vi "Calcu_Comp_Tens.vi"(8 "error in":errorcluster caption="에러 입력(에러 없음)", 9 "클러스터":T1, 10 "Condition set":string[][][](array[string]), 11 "Func_ext":string) -> (0 "error out":errorcluster caption="에러 출력", 1 "단 번호":i32, 2 "Resolution":string[][][](array[string]), 3 "Spec Out":string[][][](array[string]), 4 "ItemNames 출력":string[][](array[string]), 5 "condition out":string[][][](array[string]), 6 "cmc out":string[][][](array[string]), 7 "Spec Default":string[][][](array[string]))   [LabVIEW 2020]
uses:
  Controls/Cmd_Var Data IO.ctl
  Public/Polymorph/Data Class_2D Str.vi
  Public/Polymorph/Rmv Empt Arr_2D Str.vi
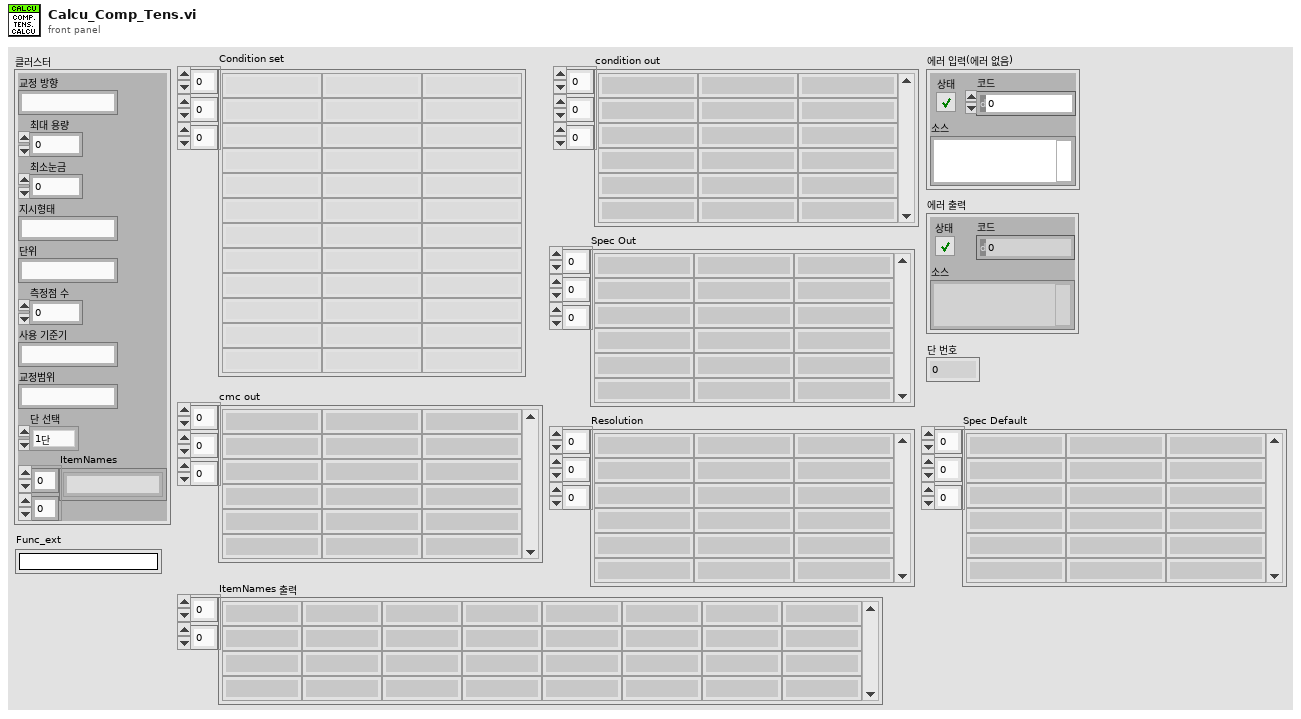
[diagram p1: front panel]
types:
  T1 = cluster{"교정 방향":string, "최대 용량":dbl, "최소눈금":dbl, "지시형태":string, "단위":string, "측정점 수":u8, "사용 기준기":string, "교정범위":string, "단 선택":enum8{"1단", "2단", "3단", "4단", "5단", "6단", "7단", "8단", "9단", "10단"}, "ItemNames":string[][]}
  T2 = typedef "Cmd_Var Data IO.ctl" = enum16{"Condition", "Condition Default", "Condition_Temp", "Resolution", "Resolution Default", "Resolution Old", "Spec", "Spec Default", "Spec Old", "Spec Temp", "Result", "Result2", "Result3", "Result_Temp", "Result_ADJ", "Result_ADJ2", "STD1", "STD2", "STD3", "STD4", "STD5", "STD Temp", "CMC", "CMC Default"}
  T3 = enum8{"1단", "2단", "3단", "4단", "5단", "6단", "7단", "8단", "9단", "10단"}
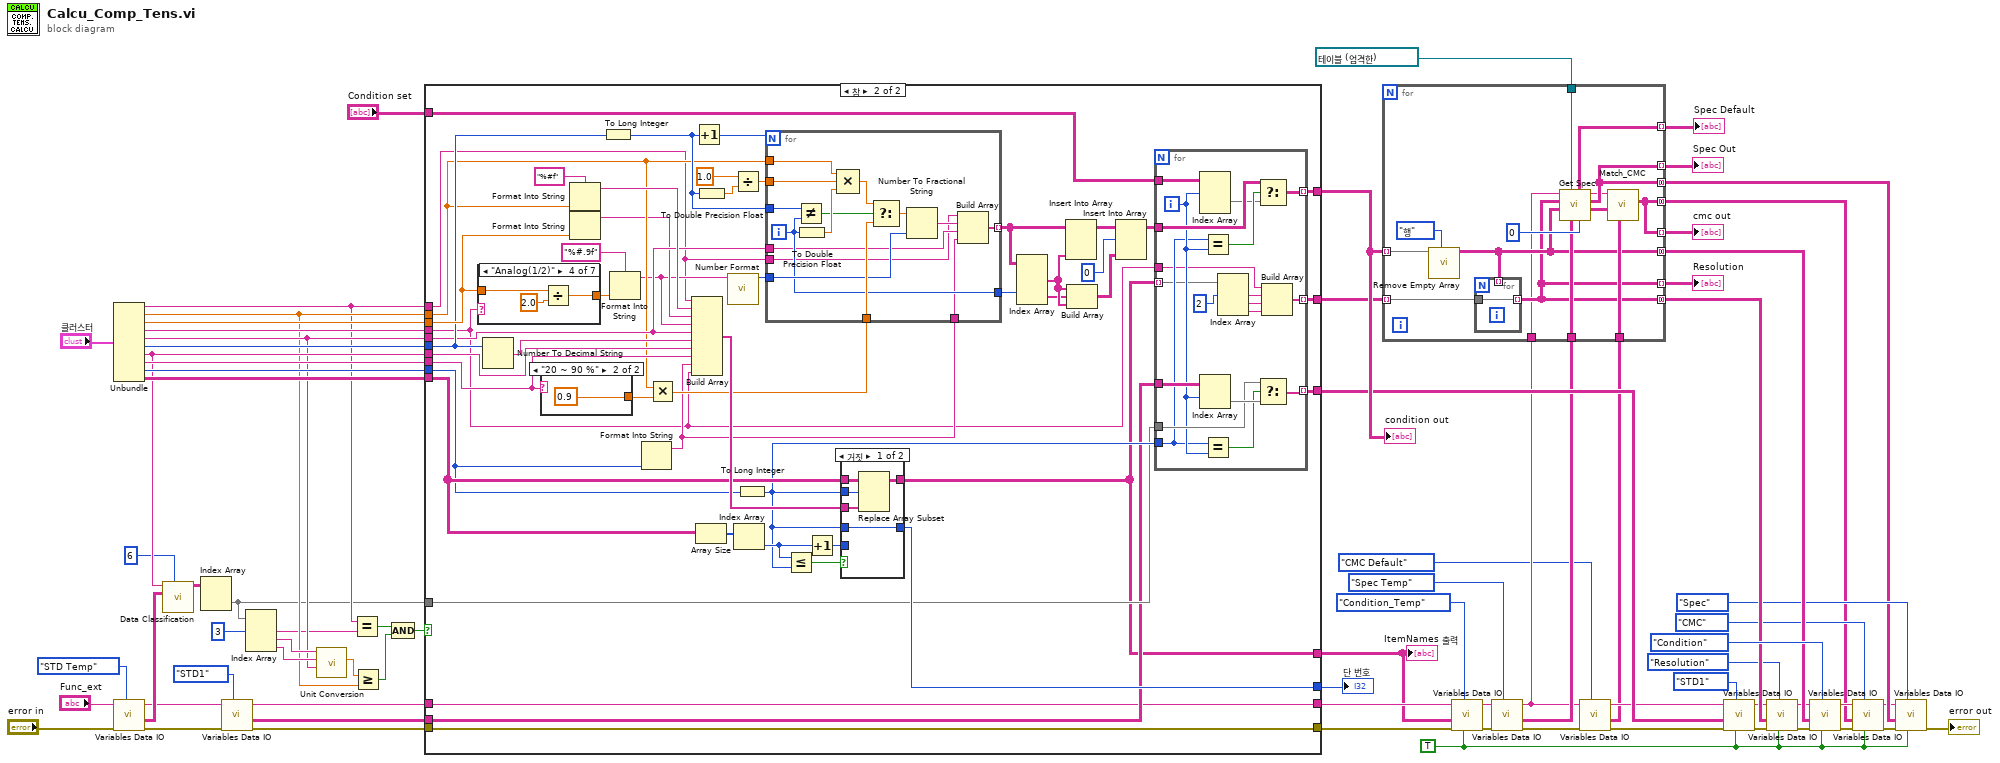
[diagram p0: block diagram]
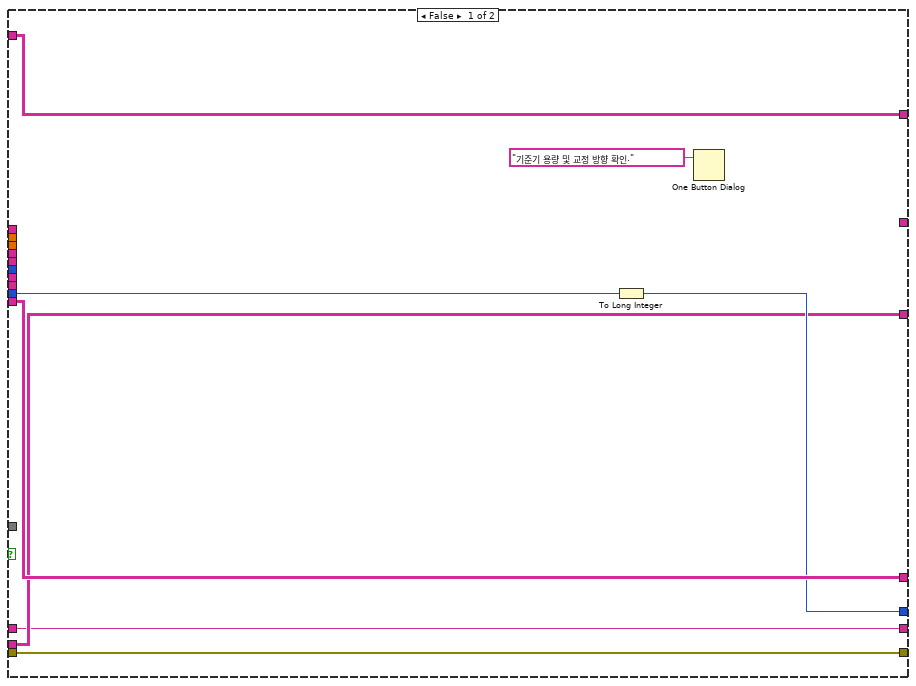
[diagram p2: hidden frame]
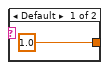
[diagram p3: hidden frame]
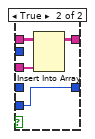
[diagram p4: hidden frame]
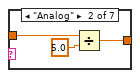
[diagram p6: hidden frame]
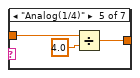
[diagram p8: hidden frame]
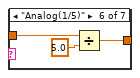
[diagram p9: hidden frame]
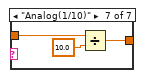
[diagram p10: hidden frame]
diagram:
  w2 = TRUE ("Write blank data ?(T)")
  n1 = Unbundle("클러스터") -> ("교정 방향"=w58:string, "최대 용량"=w60:dbl, "최소눈금"=w74:dbl, "지시형태"=w73:string, "단위"=w62:string, "측정점 수"=w70:u8, "사용 기준기"=w67:string, "교정범위"=w69:string, "단 선택"=w71:T3, "ItemNames"=w72:string[][])
  n2 = call "Variables Data IO.vi"("Select"=Cmd_Var_Data_IO."STD Temp", "error in"="error in", "Func_ext"="Func_ext") -> ("error out"=w44:errorcluster, "Data Out"=w46:string[][], "Func_ext Out"=w43:string)  [unwired: 6 in]
  n3 = call-poly "Data Classification.vi"("인덱스"=6, "DATA 입력"=w46, "검색 문자열"=w67) -> ("DATA 출력"=w66:string[][])  [unwired: 4 in, 4 out]
  n4 = Index Array(array=w66) -> (element=w53:string[])  [unwired: 2 in]
  n5 = call "Variables Data IO.vi"("Select"=Cmd_Var_Data_IO."STD1", "error in"=w44, "Func_ext"=w43) -> ("error out"=w38:errorcluster, "Data Out"=w41:string[][], "Func_ext Out"=w35:string)  [unwired: 6 in]
  n6 = Index Array(array=w53, index #1=3 ("인덱스")) -> (element #1=w59:string, element #2=w64:string, element #3=w63:string)  [unwired: 2 in]
  n7 = call "Unit Conversion.vi"("환산단위"=w62, "입력단위"=w63, "입력값"=w64) -> ("환산값 (DBL)"=w61:dbl)  [unwired: 3 in, 5 out]
  n8 = Equal?(x=w58, y=w59) -> (x = y?=w57:bool)
  n9 = Greater Or Equal?(x=w61, y=w60) -> (x >= y?=w56:bool)
  n10 = Compound Arithmetic op=AND(w57, w56) -> (w54:bool)
  n11 = case shown="참" w54 {
    tunnel: w74 -> [_ w126]
    tunnel: w73 -> [_ w84]
    tunnel: w72 -> [w82 w124]
    tunnel: w71 -> [w81 w86]
    tunnel: w70 -> [_ w123]
    tunnel: w69 -> [_ w122]
    tunnel: [w80 w106] -> w68
    tunnel: [w83 w104] -> w51
    tunnel: [w82 w89] -> w3
    tunnel: w67 -> [_ w101]
    tunnel: w62 -> [_ w100]
    tunnel: w60 -> [_ w99]
    tunnel: w58 -> [_ w87]
    tunnel: w53 -> [_ w97]
    tunnel: "Condition set" -> [w83 w98]
    tunnel: w41 -> [w79 w96]
    tunnel: [w79 w95] -> w39
    tunnel: [w77 w92] -> w8
    tunnel: w35 -> [w77 w92]
    tunnel: [w76 w93] -> w7
    tunnel: w38 -> [w76 w93]
    tunnel: [_ w88] -> w34
    frame False {
      n12 = To Long Integer(number=w81) -> (32bit integer=w80:i32)
      n13 = One Button Dialog(message="기준기 용량 및 교정 방향 확인." ("메시지")) -> ()  [unwired: 1 in, 1 out]
    }
    frame True {
      w133 = "%#f" ("포맷 문자열")
      n14 = case shown="\"Analog(1/2)\"" w84 {
        tunnel: w126 -> [w179 w182 w183 w186 w189 w192 w195]
        tunnel: [w179 w180 w183 w184 w187 w190 w193] -> w129
        frame Default {
        }
        frame "Analog" {
          n15 = Divide(x=w182, y=5.0) -> (x/y=w180:dbl)
        }
        frame "Analog(1/1)" {
        }
        frame "Analog(1/2)" {
          n16 = Divide(x=w186, y=2.0) -> (x/y=w184:dbl)
        }
        frame "Analog(1/4)" {
          n17 = Divide(x=w189, y=4.0) -> (x/y=w187:dbl)
        }
        frame "Analog(1/5)" {
          n18 = Divide(x=w192, y=5.0) -> (x/y=w190:dbl)
        }
        frame "Analog(1/10)" {
          n19 = Divide(x=w195, y=10.0) -> (x/y=w193:dbl)
        }
      }
      n20 = Number To Decimal String(number=w123) -> (decimal integer string=w130:string)  [unwired: 1 in]
      n21 = case shown="\"20 ~ 90 %\"" w122 {
        tunnel: [1.0 0.9] -> w120
        frame Default {
        }
        frame "20 ~ 90 %" {
        }
      }
      n22 = Format Into String(format string=w133, w99) -> (resulting string=w127:string)  [unwired: 2 in, 1 out]
      n23 = Format Into String(format string=w133, w126) -> (resulting string=w91:string)  [unwired: 2 in, 1 out]
      n24 = To Long Integer(number=w123) -> (32bit integer=w115:i32)
      n25 = Format Into String(format string="%#.9f" ("포맷 문자열"), w129) -> (resulting string=w90:string)  [unwired: 2 in, 1 out]
      n26 = Format Into String(w86) -> (resulting string=w85:string)  [unwired: 3 in, 1 out]
      n27 = Multiply(x=w99, y=w120) -> (x*y=w119:dbl)
      n28 = Build Array(w87, w127, w91, w90, w100, w130, w101, w122, w85, w84) -> (w131:string[])
      n29 = Increment(x=w115) -> (x+1=w121:i32)
      n30 = Array Size(array=w124) -> (size(s)=w132:i32[])
      n31 = To Double Precision Float(number=w115) -> (double precision float=w116:dbl)
      n32 = call "Number Format.vi"("입력값"=w90) -> ("정밀도(단위적용)"=w118:i32)  [unwired: 10 in]
      n33 = Divide(x=1.0, y=w116) -> (x/y=w114:dbl)
      n34 = Index Array(array=w132) -> (element=w125:i32)  [unwired: 1 in]
      n35 = To Long Integer(number=w86) -> (32bit integer=w103:i32)
      n36 = for {
        N: w121 -> [_]
        tunnel: [w160] -> w113 mode=indexing
        tunnel: w99 -> [w168]
        tunnel: w115 -> [w167]
        tunnel: w119 -> [w166]
        tunnel: w118 -> [w161]
        tunnel: w114 -> [w162]
        tunnel: w100 -> [w157]
        tunnel: [w158] -> w94
        tunnel: w87 -> [w156]
        tunnel: w85 -> [w155]
        i -> [w158]
        n37 = Not Equal?(x=w167, y=w158) -> (x != y?=w165:bool)
        n38 = To Double Precision Float(number=w158) -> (double precision float=w169:dbl)
        n39 = Compound Arithmetic op=MULTIPLY(w168, w162, w169) -> (w164:dbl)
        n40 = Select(t=w164, s=w165, f=w166) -> (s? t:f=w159:dbl)
        n41 = Number To Fractional String(number=w159, precision (6)=w161) -> (F-format string=w163:string)  [unwired: 2 in]
        n42 = Build Array(w156, w163, w157, w155) -> (w160:string[])
      }
      n43 = Less Or Equal?(x=w125, y=w103) -> (x <= y?=w107:bool)
      n44 = Increment(x=w125) -> (x+1=w105:i32)
      n45 = case shown="거짓" w107 {
        tunnel: [w173 w178] -> w89
        tunnel: w131 -> [w172 w177]
        tunnel: w124 -> [w174 w176]
        tunnel: w103 -> [w171 _]
        tunnel: w105 -> [_ w175]
        tunnel: [w170 w175] -> w106
        tunnel: w103 -> [w170 _]
        frame False {
          n46 = Replace Array Subset(array=w174, new element=w172, index (row)=w171) -> (w173:string[][])  [unwired: 1 in]
        }
        frame True {
          n47 = Insert Into Array(array=w176, new element=w177) -> (w178:string[][])  [unwired: 2 in]
        }
      }
      n48 = Index Array(array=w113, index (row) #2=w94) -> (element #1=w112:string[], element #2=w111:string[])  [unwired: 3 in]
      n49 = Insert Into Array(array=w113, new element=w112) -> (w110:string[][])  [unwired: 2 in]
      n50 = Build Array(w112, w111, w112) -> (w109:string[][])
      n51 = Insert Into Array(array=w110, index (row)=0 ("인덱스 (행)"), new element=w109) -> (w102:string[][])  [unwired: 1 in]
      n52 = for {
        tunnel: w98 -> [w150]
        tunnel: [w141] -> w104 mode=indexing
        tunnel: w103 -> [w143]
        tunnel: w102 -> [w151]
        tunnel: w97 -> [w146]
        tunnel: w96 -> [w145]
        tunnel: [w142] -> w95 mode=indexing
        tunnel: w89 -> [w140] mode=indexing
        tunnel: w84 -> [w135]
        tunnel: [w134] -> w88 mode=indexing
        i -> [w144]
        n53 = Index Array(array=w150, index (dim 0)=w144) -> (element=w149:string[][])  [unwired: 2 in]
        n54 = Index Array(array=w145, index (row)=w144) -> (element=w148:string[])  [unwired: 1 in]
        n55 = Equal?(x=w143, y=w144) -> (x = y?=w152:bool)
        n56 = Equal?(x=w143, y=w144) -> (x = y?=w147:bool)
        n57 = Index Array(array=w140, index #1=2 ("인덱스")) -> (element #1=w138:string, element #2=w137:string, element #3=w136:string)  [unwired: 2 in]
        n58 = Select(t=w151, s=w152, f=w149) -> (s? t:f=w141:string[][])
        n59 = Select(t=w146, s=w147, f=w148) -> (s? t:f=w142:string[])
        n60 = Build Array(w135, w138, w137, w136) -> (w134:string[])
      }
    }
  }
  "ItemNames 출력" <- w3
  "condition out" <- w51
  "단 번호" <- w68
  n61 = call "Variables Data IO.vi"("Write blank data ?(F)"=w2, "Select"=Cmd_Var_Data_IO."Condition_Temp", "error in"=w7, "Data In"=w3, "Func_ext"=w8) -> ("error out"=w6:errorcluster, "Func_ext Out"=w5:string)  [unwired: 4 in, 1 out]
  n62 = call "Variables Data IO.vi"("Select"=Cmd_Var_Data_IO."Spec Temp", "error in"=w6, "Func_ext"=w5) -> ("error out"=w20:errorcluster, "Data Out"=w32:string[][], "Func_ext Out"=w21:string)  [unwired: 6 in]
  n63 = call "Variables Data IO.vi"("Select"=Cmd_Var_Data_IO."CMC Default", "error in"=w20, "Func_ext"=w21) -> ("error out"=w19:errorcluster, "Data Out"=w16:string[][], "Func_ext Out"=w18:string)  [unwired: 6 in]
  n64 = for {
    tunnel: w51 -> [w210] mode=indexing
    tunnel: [w198] -> w49 mode=concatenating
    tunnel: [w197] -> w37 mode=concatenating
    tunnel: w34 -> [w208] mode=indexing
    tunnel: w21 -> [w196]
    tunnel: w32 -> [w199]
    tunnel: [w206] -> w31 mode=indexing
    tunnel: refnum<vi> refnum ("Spec Ref.") -> [w207]
    tunnel: [w206] -> w27 mode=concatenating
    tunnel: [w197] -> w22 mode=indexing
    tunnel: w16 -> [w203]
    tunnel: [w202] -> w10 mode=concatenating
    tunnel: [w202] -> w9 mode=indexing
    tunnel: [w201] -> w1 mode=indexing
    n65 = call-poly "Remove Empty Array.vi"("조건"=enum16{"행", "열", "행,열"}."행", "Data in"=w210) -> ("Data out"=w198:string[][])  [unwired: 8 in, 1 out]
    n66 = for {
      tunnel: w198 -> [_] mode=indexing
      tunnel: w208 -> [w211]
      tunnel: [w211] -> w197 mode=indexing
    }
    n67 = call "Get Spec.vi"("NumRows"=u32 0, "Spec in"=w199, "Spec Ref."=w207, "Condition in"=w198, "Resolution in"=w197, "Func_ext"=w196) -> ("Data Out"=w204:string[][], "Spec Out"=w206:string[][], "Func_ext Out"=w205:string, "Spec (Default)"=w201:string[][])  [unwired: 1 in, 1 out]
    n68 = call "Match_CMC.vi"("CMC IN"=w203, "Condition IN"=w204, "Func_ext"=w205) -> ("CMC Out"=w202:string[][])  [unwired: 5 in, 3 out]
  }
  "Spec Out" <- w31
  "Resolution" <- w22
  "cmc out" <- w9
  "Spec Default" <- w1
  n69 = call "Variables Data IO.vi"("Write blank data ?(F)"=w2, "Select"=Cmd_Var_Data_IO."STD1", "error in"=w19, "Data In"=w39, "Func_ext"=w18) -> ("error out"=w25:errorcluster, "Func_ext Out"=w26:string)  [unwired: 4 in, 1 out]
  n70 = call "Variables Data IO.vi"("Write blank data ?(F)"=w2, "Select"=Cmd_Var_Data_IO."Resolution", "error in"=w25, "Data In"=w37, "Func_ext"=w26) -> ("error out"=w24:errorcluster, "Func_ext Out"=w23:string)  [unwired: 4 in, 1 out]
  n71 = call "Variables Data IO.vi"("Write blank data ?(F)"=w2, "Select"=Cmd_Var_Data_IO."Condition", "error in"=w24, "Data In"=w49, "Func_ext"=w23) -> ("error out"=w15:errorcluster, "Func_ext Out"=w14:string)  [unwired: 4 in, 1 out]
  n72 = call "Variables Data IO.vi"("Write blank data ?(F)"=w2, "Select"=Cmd_Var_Data_IO."CMC", "error in"=w15, "Data In"=w10, "Func_ext"=w14) -> ("error out"=w13:errorcluster, "Func_ext Out"=w12:string)  [unwired: 4 in, 1 out]
  n73 = call "Variables Data IO.vi"("Write blank data ?(F)"=w2, "Select"=Cmd_Var_Data_IO."Spec", "error in"=w13, "Data In"=w27, "Func_ext"=w12) -> ("error out"=→"error out":errorcluster)  [unwired: 4 in, 2 out]
